vi "PCO_OpenCameraEx.vi"(8 "error in (no error)":errorcluster {"code" format="%x"}, 10 "strOpenStruct":T1 {"wInterfaceType" format="%x"}) -> (0 "error out":errorcluster {"code" format="%x"}, 2 "ErrorMessage":i32 format="%x", 3 "ph out":u64)   [LabVIEW 2019, in "SDK.lvlib" / "CameraAccess.lvlib"]
doc: "<b>Description:</b>\nThis function is used to get a connection to a distinct camera, e.g. a camera which is connected to a specific interface port. A unique handle is returned, which must be used for all other function calls. To select the desired camera the structure PCO_Openstruct structure must be filled with appropriate parameters before the function is called. If no camera could be found at the selected interface an error is returned and the handle is set to NULL.\n\nAs a special case this function can be used to establish a valid connection to a camera through the serial interface of any Camera Link grabber to control the camera with the PCO SDK functions. The image grab and transfer functions of the pco.sdk can not be used in this mode. The name of the grabber manufacturer clserxxx.dll must be provided in the PCO_Openstruct structure.\n\nIf more then one camera with GigE interface are used, only those cameras can be opened, which have established a connection with a valid IP address, when the PCO_OpenCameraEx function is called the first time from an application.\n\n<b>Supported camera type:</b>\nAll cameras\n\n<b>Descriptor dependency:</b>\nNone"
uses:
  CameraAccess.lvlib
  Structures/Structures.lvlib
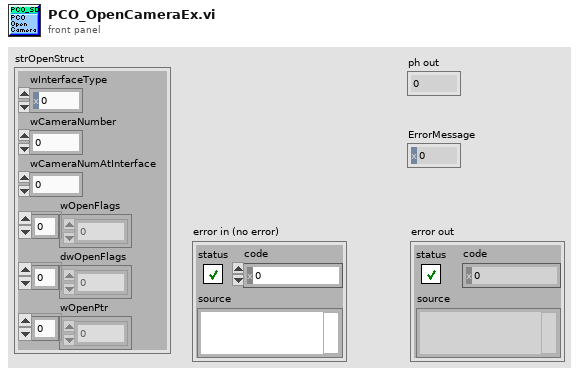
[diagram p1: front panel]
types:
  T1 = cluster{"wInterfaceType":u16, "wCameraNumber":u16, "wCameraNumAtInterface":u16, "wOpenFlags":u16[], "dwOpenFlags":u32[], "wOpenPtr":u64[]}
  T2 = cluster{"wSize":u16, "wInterfaceType":u16, "wCameraNumber":u16, "wCameraNumAtInterface":u16, "wOpenFlags":cluster{u16, u16, u16, u16, u16, u16, u16, u16, u16, u16}, "dwOpenFlags":cluster{u32, u32, u32, u32, u32}, "wOpenPtr":cluster{u64, u64, u64, u64, u64, u64}, "zzWDummy":cluster{u16, u16, u16, u16, u16, u16, u16, u16}}
  T3 = cluster{"wSize":u16, "wInterfaceType":u16, "wCameraNumber":u16, "wCameraNumAtInterface":u16, "wOpenFlags":cluster{u16, u16, u16, u16, u16, u16, u16, u16, u16, u16}, "dwOpenFlags":cluster{u32, u32, u32, u32, u32}, "wOpenPtr":cluster{u32, u32, u32, u32, u32, u32}, "zzWDummy":cluster{u16, u16, u16, u16, u16, u16, u16, u16}}
  T4 = cluster{"wOpenFlags[0]":u16, "wOpenFlags[1]":u16, "wOpenFlags[2]":u16, "wOpenFlags[3]":u16, "wOpenFlags[4]":u16, "wOpenFlags[5]":u16, "wOpenFlags[6]":u16, "wOpenFlags[7]":u16, "wOpenFlags[8]":u16, "wOpenFlags[9]":u16}
  T5 = cluster{"dwOpenFlags[0]":u32, "dwOpenFlags[1]":u32, "dwOpenFlags[2]":u32, "dwOpenFlags[3]":u32, "dwOpenFlags[4]":u32}
  T6 = cluster{"wOpenPtr[0]":u64, "wOpenPtr[1]":u64, "wOpenPtr[2]":u64, "wOpenPtr[3]":u64, "wOpenPtr[4]":u64, "wOpenPtr[5]":u64}
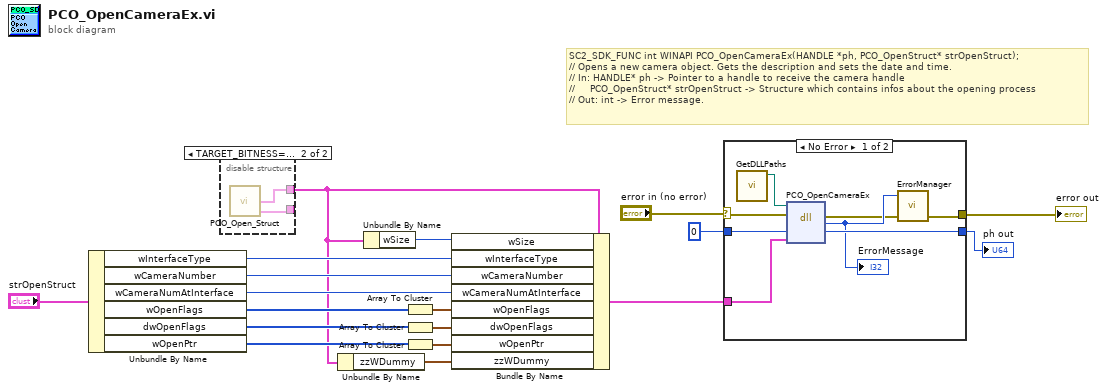
[diagram p0: block diagram]
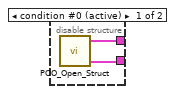
[diagram p2: hidden frame]
diagram:
  # "SC2_SDK_FUNC int WINAPI PCO_OpenCameraEx(HANDLE *ph, PCO_OpenStruct* strOpenStruct);\n// Opens a new camera object. Gets the description and sets the date and time.\n// In: HANDLE* ph -> Pointer to a handle to receive the camera handle\n//     PCO_OpenStruct* strOpenStruct -> Structure which contains infos about the opening process\n// Out: int -> Error message."
  n1 = Unbundle By Name("strOpenStruct") -> ("wInterfaceType"=w11:u16, "wCameraNumber"=w10:u16, "wCameraNumAtInterface"=w9:u16, "wOpenFlags"=w8:u16[], "dwOpenFlags"=w5:u32[], "wOpenPtr"=w6:u64[])
  n2 = disable-structure "Diagram Disable Structure" shown="TARGET_BITNESS==32" {
    disable-tunnel: [w20 w22] -> w2
    disable-tunnel: [w19 w21] -> _
    frame condition #0 (active) {
      n3 = call "PCO_Open_Struct.vi"() -> ("PCO_OpenStruct_Raw_x64"=w20:T2, "PCO_Open_Struct"=w19:T1)  [unwired: 4 in, 3 out]
    }
    frame condition #1 {
      n4 = call "PCO_Open_Struct.vi"() -> ("PCO_OpenStruct_Raw_win32"=w22:T3, "PCO_Open_Struct"=w21:T1)  [unwired: 4 in, 3 out]
    }
  }
  n5 = Unbundle By Name(w2) -> ("zzWDummy"=w1:cluster{u16, u16, u16, u16, u16, u16, u16, u16})
  n6 = Unbundle By Name(w2) -> ("wSize"=w12:u16)
  n7 = Array To Cluster(array=w8) -> (cluster=w7:T4)
  n8 = Array To Cluster(array=w5) -> (cluster=w4:T5)
  n9 = Array To Cluster(array=w6) -> (cluster=w3:T6)
  n10 = Bundle By Name(cluster=w2, "wSize"=w12, "wInterfaceType"=w11, "wCameraNumber"=w10, "wCameraNumAtInterface"=w9, "wOpenFlags"=w7, "dwOpenFlags"=w4, "wOpenPtr"=w3, "zzWDummy"=w1) -> (w13:T2)
  n11 = case shown="No Error" "error in (no error)" {
    selector: "error in (no error)" -> [w30 w31]
    tunnel: [w25 w31] -> w18
    tunnel: w13 -> [w24 _]
    tunnel: u64 0 ("ph") -> [w29 w32]
    tunnel: [w28 w32] -> w16
    frame No Error {
      n12 = call "GetDLLPaths.vi"() -> ("SC2_Cam_Path"=w23:path)  [unwired: 9 in, 2 out]
      n13 = dll-call lib="?" fn="PCO_OpenCameraEx"(path in=w23, error in=w30, "ph"=w29, "strOpenStruct"=w24) -> (error out=w26:errorcluster, "ErrorMessage"=w27:i32, "ph"=w28:u64)  [unwired: 2 in, 1 out]
      "ErrorMessage" <- w27
      n14 = call "ErrorManager.vi"("error in (no error)"=w26, "error code"=w27) -> ("error out"=w25:errorcluster)  [unwired: 3 in]
    }
    frame Error {
    }
  }
  "error out" <- w18
  "ph out" <- w16
